vi "File5Info.vi"(9 "Language":u32, 10 "TypeIn":string, 11 "file path (dialog if empty)":path) -> (0 "ModificationTimeOut":string, 1 "FileSizeOut":string, 2 "DirectoryOut":string, 3 "FileNameOut":string, 4 "FileTypeOut":string)   [LabVIEW 2015]
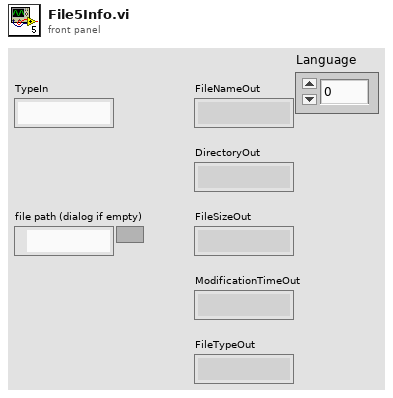
[diagram p1: front panel]
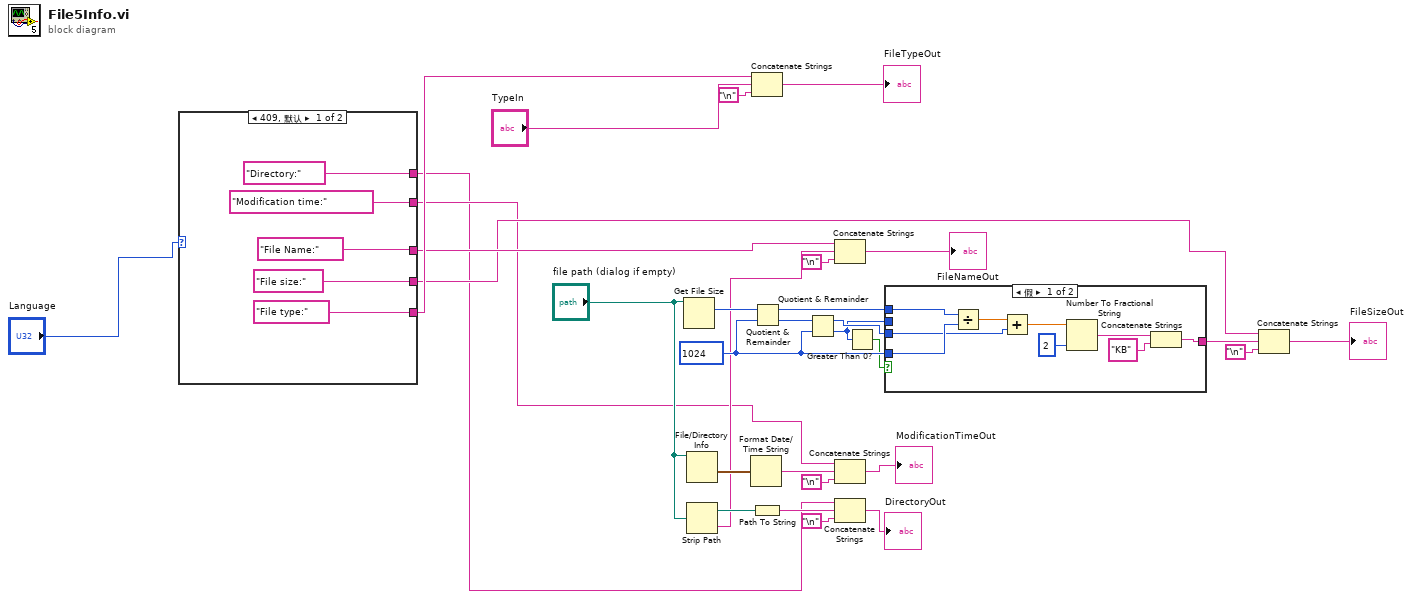
[diagram p0: block diagram]
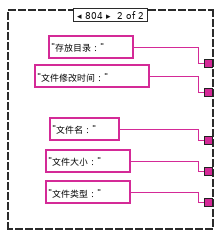
[diagram p2: hidden frame]
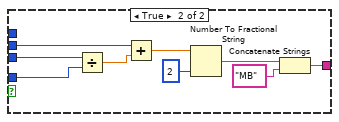
[diagram p3: hidden frame]
diagram:
  w18 = i64 1024 ("y")
  n1 = case shown="409, 默认" "Language" {
    tunnel: ["Modification time:" "文件修改时间："] -> w2
    tunnel: ["Directory:" "存放目录："] -> w1
    tunnel: ["File Name:" "文件名："] -> w4
    tunnel: ["File size:" "文件大小："] -> w3
    tunnel: ["File type:" "文件类型："] -> w5
    frame 409, Default {
    }
    frame 804 {
    }
  }
  n2 = Get File Size(file="file path (dialog if empty)") -> (size (in bytes)=w15:i64)  [unwired: 1 in, 2 out]
  n3 = File/Directory Info(path="file path (dialog if empty)") -> (last mod=w27:timestamp)  [unwired: 1 in, 6 out]
  n4 = Strip Path(path="file path (dialog if empty)") -> (stripped path=w25:path, name=w8:string)
  n5 = Format Date/Time String(seconds (now)=w27) -> (date/time string=w29:string)  [unwired: 2 in]
  n6 = Concatenate Strings(w5, "TypeIn", "\n") -> (→"FileTypeOut":string)
  n7 = Path To String(path=w25) -> (string=w24:string)
  n8 = Quotient & Remainder(x=w15, y=w18) -> (x-y*floor(x/y)=w22:i64, floor(x/y)=w16:i64)
  n9 = Quotient & Remainder(x=w16, y=w18) -> (x-y*floor(x/y)=w20:i64, floor(x/y)=w19:i64)
  n10 = Concatenate Strings(w4, w8, "\n") -> (→"FileNameOut":string)
  n11 = Concatenate Strings(w2, w29, "\n") -> (→"ModificationTimeOut":string)
  n12 = Concatenate Strings(w1, w24, "\n") -> (→"DirectoryOut":string)
  n13 = Greater Than 0?(x=w19) -> (x > 0?=w17:bool)
  n14 = case shown="假" w17 {
    tunnel: w18 -> [w47 w57]
    tunnel: w19 -> [_ w55]
    tunnel: w20 -> [w45 w58]
    tunnel: [w50 w53] -> w21
    tunnel: w22 -> [w48 _]
    frame False {
      n15 = Divide(x=w48, y=w47) -> (x/y=w46:dbl)
      n16 = Add(x=w46, y=w45) -> (x+y=w44:dbl)
      n17 = Number To Fractional String(number=w44, precision (6)=i16 2 ("精度(6)")) -> (F-format string=w42:string)  [unwired: 2 in]
      n18 = Concatenate Strings(w42, "KB" ("字符串")) -> (w50:string)
    }
    frame True {
      n19 = Divide(x=w58, y=w57) -> (x/y=w56:dbl)
      n20 = Add(x=w55, y=w56) -> (x+y=w54:dbl)
      n21 = Number To Fractional String(number=w54, precision (6)=i16 2 ("精度(6)")) -> (F-format string=w52:string)  [unwired: 2 in]
      n22 = Concatenate Strings(w52, "MB") -> (w53:string)
    }
  }
  n23 = Concatenate Strings(w3, w21, "\n") -> (→"FileSizeOut":string)
